vi "Change FromToWave_or_Time.vi"(6 "ChangeAll":bool, 7 "Combo Box":T1="Spectra", 8 "error in (no error)":errorcluster, 9 "To":dbl, 10 "From":dbl, 11 "Control-Client in":refnum<class "Control-Client.lvclass">) -> (0 "error out":errorcluster, 3 "Control-Client out":refnum<class "Control-Client.lvclass">)   [LabVIEW 2018, in "Control-Client.lvclass"]
uses:
  Control-Client.lvclass
  dependecies/ControlsVIs/Clusters-def/Types_of_Graphs-Client.ctl
  Control-Client.lvclass/Control-Client.ctl
  Experiments/Experiment.lvclass
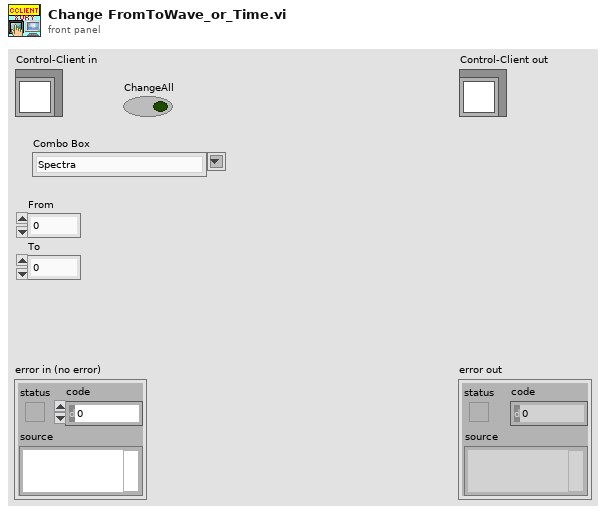
[diagram p1: front panel]
types:
  T1 = typedef "Control-Client.lvclass/Types_of_Graphs-Client.ctl" = string
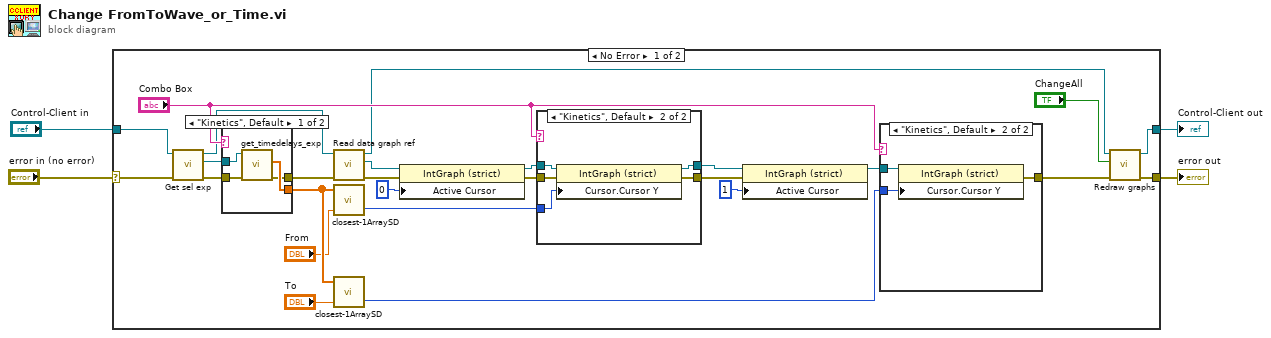
[diagram p0: block diagram]
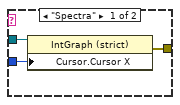
[diagram p2: hidden frame]
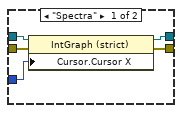
[diagram p3: hidden frame]
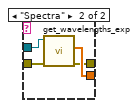
[diagram p4: hidden frame]
diagram:
  n1 = case shown="No Error" "error in (no error)" {
    selector: "error in (no error)" -> [w10 w56]
    tunnel: [w17 w56] -> w3
    tunnel: [w16 w55] -> w1
    tunnel: "Control-Client in" -> [w6 w55]
    frame No Error {
      n2 = call "Get sel exp.vi"("error in (no error)"=w10, "Control-Client in"=w6) -> ("error out"=w11:errorcluster, "Sel experiment"=w12:refnum<class "Experiment.lvclass">, "Control-Client out"=w8:refnum<class "Control-Client.lvclass">)  [unwired: 7 in]
      n3 = case shown="\"Kinetics\", Default" "Combo Box" {
        tunnel: [w48 w54] -> w30
        tunnel: w12 -> [w50 w53]
        tunnel: w11 -> [w49 w52]
        tunnel: [w47 w51] -> w9
        frame "Kinetics", Default {
          n4 = call "get_timedelays_exp.vi"("error in (no error)"=w49, "Experiment.lvclass in"=w50) -> ("error out"=w47:errorcluster, "timedelays"=w48:dbl[])  [unwired: 7 in, 1 out]
        }
        frame "Spectra" {
          n5 = call "get_wavelengths_exp.vi"("error in (no error)"=w52, "Experiment.lvclass in"=w53) -> ("error out"=w51:errorcluster, "wavelengths"=w54:dbl[])  [unwired: 7 in, 1 out]
        }
      }
      n6 = call "Read data graph ref.vi"("error in (no error)"=w9, "Control-Client in"=w8) -> ("error out"=w21:errorcluster, "Exp data graph ref"=w22:refnum<vi>, "Control-Client out"=w7:refnum<class "Control-Client.lvclass">)  [unwired: 7 in]
      n7 = call "closest-1ArraySD.vi"("desired element"="From", "1D Array"=w30) -> ("closest index"=w15:i32)  [unwired: 1 in, 1 out]
      n8 = call "closest-1ArraySD.vi"("desired element"="To", "1D Array"=w30) -> ("closest index"=w14:i32)  [unwired: 1 in, 1 out]
      n9 = property class="IntGraph (strict)"(reference=w22, error in=w21, "Active Cursor"=u32 0) -> (reference out=w29:refnum<vi>, error out=w20:errorcluster)
      n10 = case shown="\"Kinetics\", Default" "Combo Box" {
        tunnel: w29 -> [w41 w46]
        tunnel: [w40 w45] -> w28
        tunnel: w15 -> [w39 w44]
        tunnel: w20 -> [w38 w43]
        tunnel: [w37 w42] -> w19
        frame "Spectra" {
          n11 = property class="IntGraph (strict)"(reference=w41, error in=w38, "Cursor.Cursor X"=w39) -> (reference out=w40:refnum<vi>, error out=w37:errorcluster)
        }
        frame "Kinetics", Default {
          n12 = property class="IntGraph (strict)"(reference=w46, error in=w43, "Cursor.Cursor Y"=w44) -> (reference out=w45:refnum<vi>, error out=w42:errorcluster)
        }
      }
      n13 = property class="IntGraph (strict)"(reference=w28, error in=w19, "Active Cursor"=u32 1) -> (reference out=w27:refnum<vi>)  [unwired: 1 out]
      n14 = case shown="\"Kinetics\", Default" "Combo Box" {
        tunnel: w27 -> [w33 w36]
        tunnel: w14 -> [w32 w35]
        tunnel: [w31 w34] -> w5
        frame "Spectra" {
          n15 = property class="IntGraph (strict)"(reference=w33, "Cursor.Cursor X"=w32) -> (error out=w31:errorcluster)  [unwired: 1 in, 1 out]
        }
        frame "Kinetics", Default {
          n16 = property class="IntGraph (strict)"(reference=w36, "Cursor.Cursor Y"=w35) -> (error out=w34:errorcluster)  [unwired: 1 in, 1 out]
        }
      }
      n17 = call "Redraw graphs.vi"("error in (no error)"=w5, "ChangeAll"="ChangeAll", "Control-Client in"=w7) -> ("error out"=w17:errorcluster, "Control-Client out"=w16:refnum<class "Control-Client.lvclass">)  [unwired: 7 in]
    }
    frame Error {
    }
  }
  "error out" <- w3
  "Control-Client out" <- w1
